vi "Copy Selection.vi"   [LabVIEW 2023]
doc: "Demonstrates the Copy Selection method in VI Scripting, which places the selected portion of a VI on the system clipboard. It has the same effect as choosing Edit > Copy from the user interface."
panel:
  # "Overview: Demonstrates the Copy Selection method in VI Scripting, which places the selected portion of a VI on the system clipboard.\nInstructions:\n1. Open the front panel of Test - Selection List Target.vi.\n2. Select one or more objects.\n3. Run this VI. The selected objects will be copied to the system clipboard.\n4. Open a new VI front panel.\n5. Select Edit > Paste from the menu bar. The items you originally selected (which were programmatically copied to the clipboard) will be pasted onto the new VI front panel."
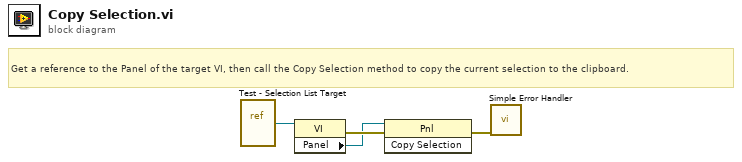
[diagram p0: block diagram]
diagram:
  # "Get a reference to the Panel of the target VI, then call the Copy Selection method to copy the current selection to the clipboard."
  n1 = vi-ref "Test - Selection List Target.vi"() -> (w4:refnum<vi>)
  n2 = property class="VI"(reference=w4) -> (error out=w3:errorcluster, "Panel"=w2:refnum<vi>)  [unwired: 1 in, 1 out]
  n3 = invoke class="Pnl" method="Copy Selection"(reference=w2, error in=w3) -> (error out=w1:errorcluster)  [unwired: 1 in, 2 out]
  n4 = call <vilib>:"Simple Error Handler.vi"("error in (no error)"=w1) -> ()  [unwired: 4 in, 5 out]
